vi "Measure all Channel Powers.vi"(8 "error in (no error)":errorcluster, 11 "2936r in":refnum<class "2936r.lvclass">) -> (0 "error out":errorcluster, 2 "Measured Power":dbl[](array[numeric]), 3 "2936r out":refnum<class "2936r.lvclass">)   [LabVIEW 2018, in "2936r.lvlib" / "2936r.lvclass"]
uses:
  2936r.lvclass
  2936r.lvclass/2936r.ctl
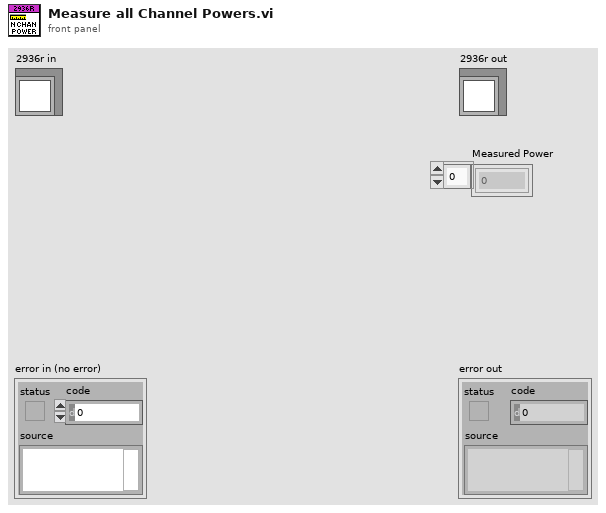
[diagram p1: front panel]
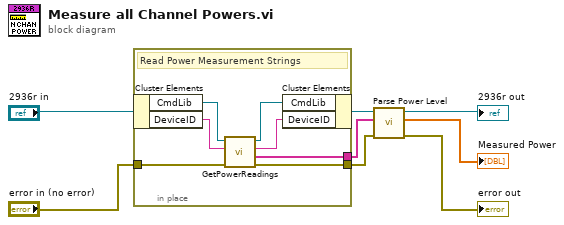
[diagram p0: block diagram]
diagram:
  n1 = in-place {
    in-place-border: [w11] -> w3
    in-place-border: "error in (no error)" -> [w10]
    in-place-border: [w9] -> w1
    # "Read Power Measurement Strings"
    n2 = in-place-cluster #1("2936r in") -> ("CmdLib"=w15:refnum<k24>, "DeviceID"=w13:string)
    n3 = call <instrlib>:"GetPowerReadings.vi"("error in"=w10, "Device Key In"=w13, "PM Cmds In"=w15) -> ("error out"=w9:errorcluster, "Power Readings"=w11:string[], "Device Key Out"=w12:string, "PM Cmds Out"=w14:refnum<k24>)  [unwired: 1 in]
    n4 = in-place-cluster #1("CmdLib"=w14, "DeviceID"=w12) -> (w4:refnum<class "2936r.lvclass">)
  }
  n5 = call "Parse Power Level.vi"("error in"=w1, "Read Values"=w3, "2936r in"=w4) -> ("error out"=→"error out":errorcluster, "Power (W)"=→"Measured Power":dbl[], "2936r out"=→"2936r out":refnum<class "2936r.lvclass">)  [unwired: 6 in]
